vi "Wait for Acquisition Complete.vi"(8 "error in (no error)":errorcluster, 9 "Maximum Time (10000 ms)":u32=10000, 11 "VISA resource name":refnum<visa-resource-name>) -> (0 "error out":errorcluster, 3 "VISA resource name out":refnum<visa-resource-name>)   [LabVIEW 2018, in "Counter.lvlib" / "PICOTEST U62XXA series.lvlib"]
doc: "Ensures that the Counter has completed all operations before a query for data is sent. This VI should be called after Initiate and before Fetch."
uses:
  PICOTEST U62XXA series.lvlib
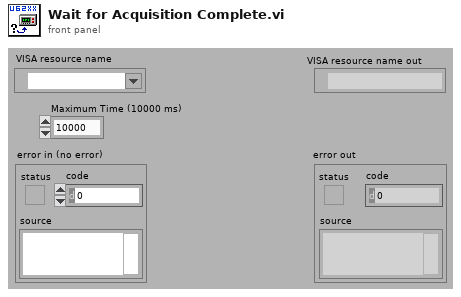
[diagram p1: front panel]
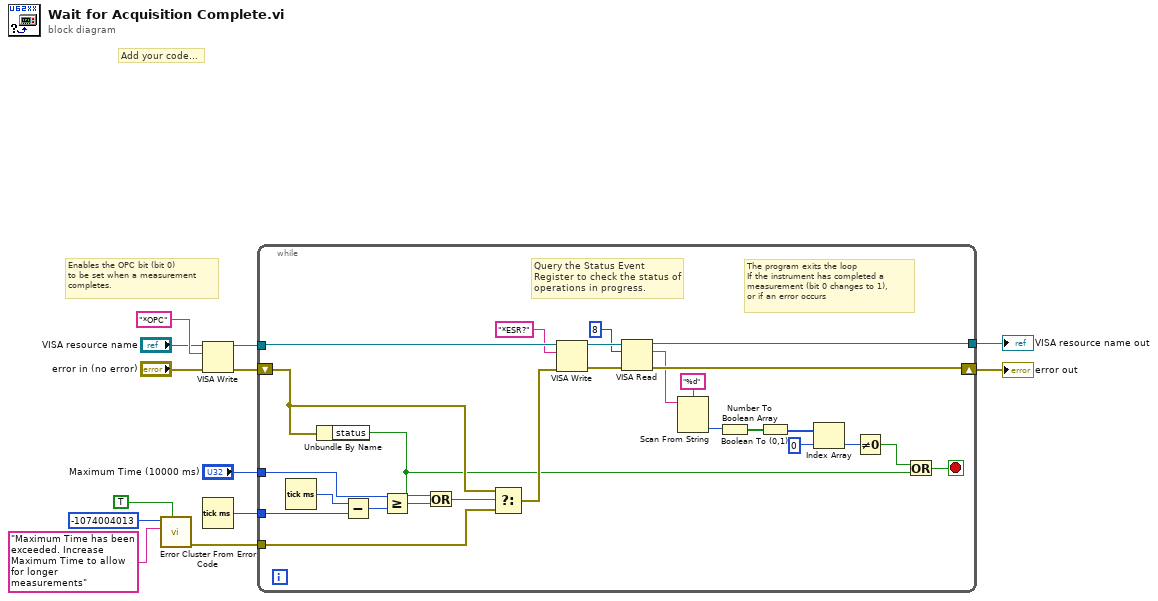
[diagram p0: block diagram]
diagram:
  # "Enables the OPC bit (bit 0)\nto be set when a measurement\ncompletes."
  # "Add your code..."
  n1 = call <vilib>:"Error Cluster From Error Code.vi"("show call chain? (False)"=TRUE, "error message (\"\")"="Maximum Time has been exceeded. Increase Maximum Time to allow for longer measurements", "error code (0)"=-1074004013) -> ("error out"=w3:errorcluster)  [unwired: 6 in]
  n2 = VISA Write(VISA resource name="VISA resource name", write buffer="*OPC", error in (no error)="error in (no error)") -> (VISA resource name out=w2:refnum<visa-resource-name>, error out=w12:errorcluster)  [unwired: 1 out]
  n3 = Tick Count (ms)() -> (millisecond timer value=w5:u32)
  n4 = while {
    tunnel: w2 -> [w26]
    tunnel: [w27] -> w11
    tunnel: w5 -> [w36]
    tunnel: "Maximum Time (10000 ms)" -> [w34]
    tunnel: w3 -> [w25]
    shift-right: [w39] -> w10
    shift-left: w12 -> [w32]
    stop <- w38 stop-if-true
    # "Query the Status Event\nRegister to check the status of\noperations in progress."
    # "The program exits the loop\nIf the instrument has completed a\nmeasurement (bit 0 changes to 1),\nor if an error occurs"
    n5 = Tick Count (ms)() -> (millisecond timer value=w35:u32)
    n6 = Unbundle By Name(w32) -> ("status"=w28:bool)
    n7 = Subtract(x=w35, y=w36) -> (x-y=w33:u32)
    n8 = Greater Or Equal?(x=w34, y=w33) -> (x >= y?=w30:bool)
    n9 = Or(x=w28, y=w30) -> (x .or. y?=w29:bool)
    n10 = Select(t=w32, s=w29, f=w25) -> (s? t:f=w31:errorcluster)
    n11 = VISA Write(VISA resource name=w26, write buffer="*ESR?", error in (no error)=w31) -> (VISA resource name out=w23:refnum<visa-resource-name>, error out=w22:errorcluster)  [unwired: 1 out]
    n12 = VISA Read(VISA resource name=w23, byte count=u32 8, error in (no error)=w22) -> (VISA resource name out=w27:refnum<visa-resource-name>, read buffer=w20:string, error out=w39:errorcluster)  [unwired: 1 out]
    n13 = Scan From String(format string="%d", input string=w20) -> (output 1=w15:i32)  [unwired: 3 in, 3 out]
    n14 = Number To Boolean Array(number=w15) -> (Boolean array=w18:bool[])
    n15 = Boolean To (0,1)(Boolean=w18) -> (0, 1=w17:i16[])
    n16 = Index Array(array=w17, index=0) -> (element=w14:i16)
    n17 = Not Equal To 0?(x=w14) -> (x != 0?=w37:bool)
    n18 = Or(x=w37, y=w28) -> (x .or. y?=w38:bool)
  }
  "VISA resource name out" <- w11
  "error out" <- w10
